vi "Get BLISS_Validate Server List.vi"(10 "Server Names":string[](array[string])) -> (3 "Enable/Disable":T1(ring))   [LabVIEW 2020]
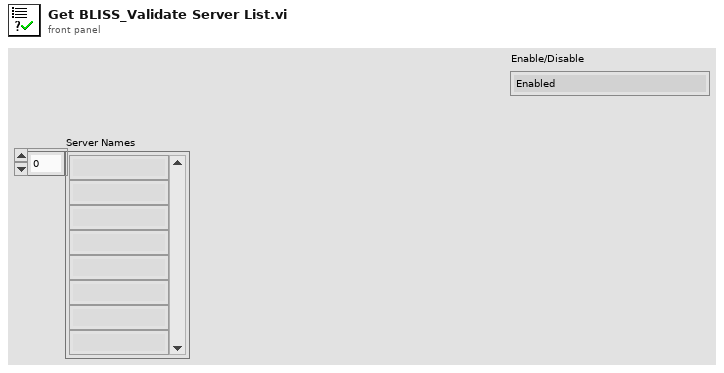
[diagram p1: front panel]
types:
  T1 = enum8{"Enabled", "Disabled", "Disabled and Grayed Out"}
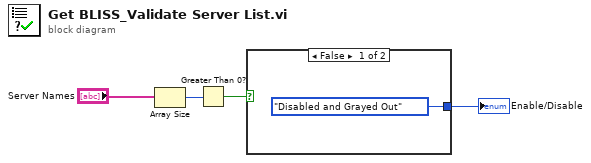
[diagram p0: block diagram]
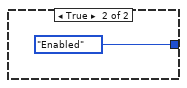
[diagram p2: hidden frame]
diagram:
  n1 = Array Size(array="Server Names") -> (size(s)=w3:i32)
  n2 = Greater Than 0?(x=w3) -> (x > 0?=w2:bool)
  n3 = case shown="False" w2 {
    tunnel: [T1."Disabled and Grayed Out" ("Disabled") T1."Enabled" ("Disabled")] -> w4
    frame False {
    }
    frame True {
    }
  }
  "Enable/Disable" <- w4
